vi "aft_LMS_Set_Memory.vi"(8 "error in":errorcluster, 10 "fixed-point LMS settings":T1, 11 "diagram":refnum<vi>) -> (0 "error out":errorcluster, 3 "diagram out":refnum<vi>)   [LabVIEW 2017, in "NI_AdaptiveFilter.lvlib"]
uses:
  <vilib>/addons/Adaptive Filters/NI_AdaptiveFilter.lvlib
  <vilib>/fxp/LVFixedPointRepBitsTypeDef.ctl
  <vilib>/rvi/ClientSDK/Core/Script/Memory/ProjectItem/Public/nirviPiMemoryType_ArbitrationOption.ctl
  <vilib>/rvi/DataTransferAndStorage/Container/Common/niFpgaContainerMemoryLatencyControl.ctl
  <vilib>/rvi/ClientSDK/Core/Script/Memory/ProjectItem/Private/nirviPiMemory_CommitLocal.vi
  <vilib>/rvi/ClientSDK/Core/Script/Memory/ProjectItem/Private/nirviPiMemory_SetArbitrationOptions.vi
  <vilib>/rvi/ClientSDK/Core/Script/Memory/ProjectItem/Private/nirviPiMemory_SetInitData2.vi
  <vilib>/rvi/ClientSDK/Core/Script/Memory/ProjectItem/Private/nirviPiMemory_SetSize.vi
  <vilib>/rvi/ClientSDK/Core/Script/Memory/ProjectItem/Private/nirviPiMemory_SetMemoryLatency.vi
  <vilib>/rvi/ClientSDK/Core/Script/Memory/ProjectItem/Private/nirviPiMemory_SetDataType2.vi
  <vilib>/rvi/ClientSDK/Core/Script/Memory/ProjectItem/Private/nirviPiMemory_OpenWithNodeRefnum.vi
  <vilib>/Utility/VariantDataType/VariantType.lvlib
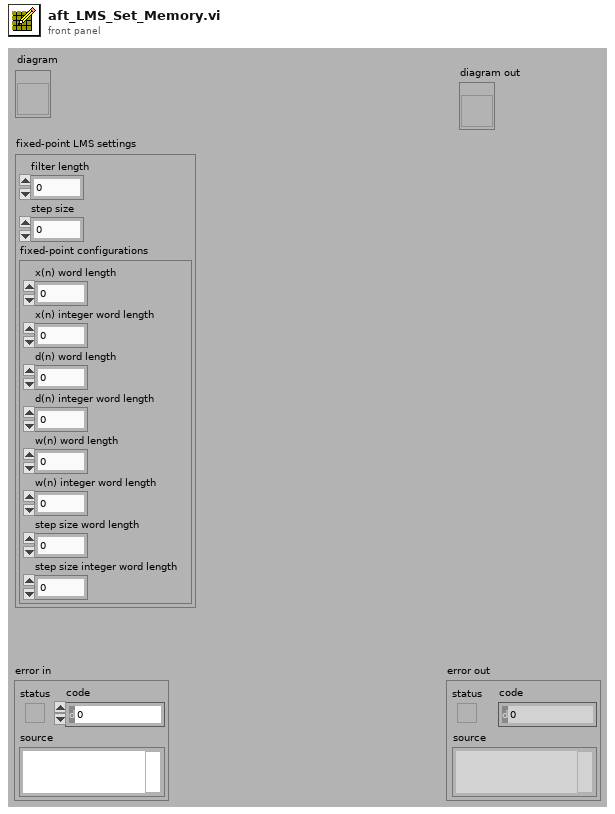
[diagram p1: front panel]
types:
  T1 = cluster{"filter length":i32, "step size":dbl, "fixed-point configurations":cluster{"x(n) word length":i32, "x(n) integer word length":i32, "d(n) word length":i32, "d(n) integer word length":i32, "w(n) word length":i32, "w(n) integer word length":i32, "step size word length":i32, "step size integer word length":i32}}
  T2 = typedef "LVFixedPointRepBitsTypeDef.ctl" = cluster{"Signed":bool, "Word Length":u32, "Integer Word Length":i32}
  T3 = typedef "nirviPiMemoryType_ArbitrationOption.ctl" = u16
  T4 = typedef "nirviPiMemory_State.ctl" = cluster{"Item":refnum<vi>, "Memory Block":T5, "Dirty":bool, "XNode":refnum<vi>, "Init Data String":string}
  T5 = typedef "niFpgaContainerState.ctl" = cluster{"displayName":string, "hardwareName":string, "dataType":T6, "elementTypeDescriptor":variant, "terminalTypeDescriptor":variant, "requestedNumberOfElements":u32, "memoryType":T7, "arbitrationForInterfaceA":T8, "numberOfElementsPerRead":u32, "arbitrationForInterfaceB":T8, "numberOfElementsPerWrite":u32, "VI_Defined":bool, "type":T9, "initializationParameters":T10, "disableOnOverflow/Underflow":bool, "interfaceConfiguration":T11, "controlLogic":T12, "actualNumberOfElements":u32, "dramSelection":string, "dramMaxOustandingRequests":i32, "dramIncludeByteEnables":bool, "dramGrantTime":u32, "fullEmulation":bool, "memoryInMultipleClockDomains":bool, "memoryLatency":T13}
  T6 = typedef "niFpgaDataTypeControl.ctl" = enum32{"Boolean", "I8", "I16", "I32", "I64", "U8", "U16", "U32", "U64", "FXP", "CustomControl", "SGL"}
  T7 = typedef "niFpgaContainerImplementationControl.ctl" = enum16{"Flip-Flops", "Look-Up Table", "Block Memory", "DRAM"}
  T8 = typedef "niFpgaContainerArbitrationOptionsControl.ctl" = enum16{"Always Arbitrate", "Arbitrate if Multiple Requestors Only", "Never Arbitrate"}
  T9 = typedef "niFpgaTransferTypeControl.ctl" = enum16{"Target-Scoped", "Host to Target - DMA", "Target to Host - DMA", "Peer to Peer Reader", "Peer to Peer Writer", "Bidirectional"}
  T10 = typedef "niFpgaContainerInitializationParameters.ctl" = cluster{"initialized":bool, "VI_Path":path, "initialData":variant}
  T11 = typedef "niFpgaMemoryInterfaceConfiguration.ctl" = enum16{"Read A-Write B", "Read A-Read B"}
  T12 = typedef "niFpgaFifoControlLogicControl.ctl" = enum16{"Slice Fabric", "Target Optimal", "Built-in"}
  T13 = typedef "niFpgaContainerMemoryLatencyControl.ctl" = u16
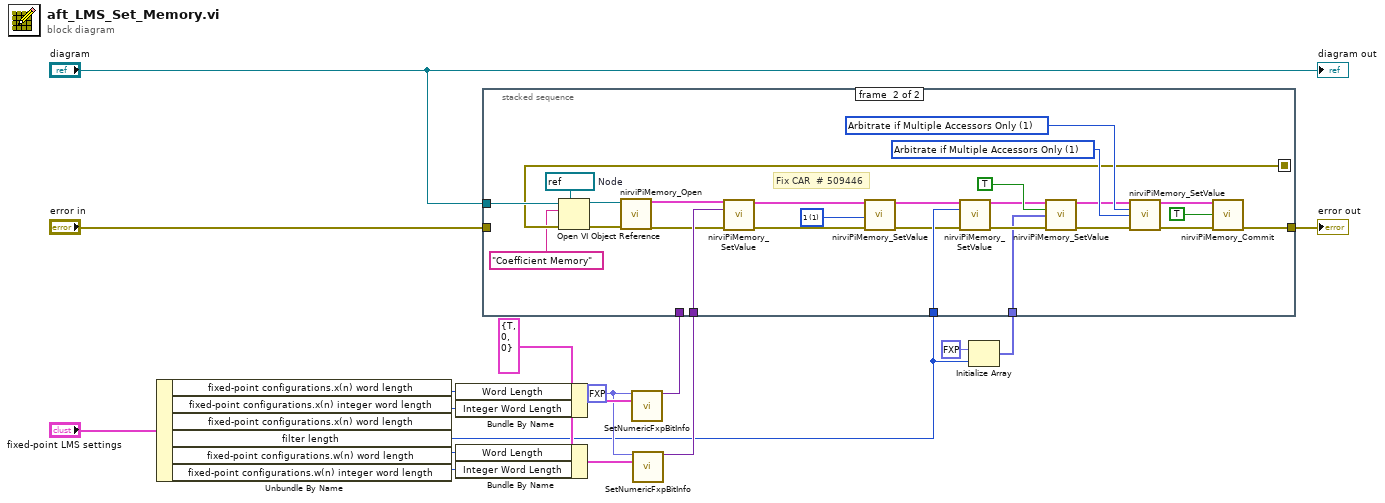
[diagram p0: block diagram]
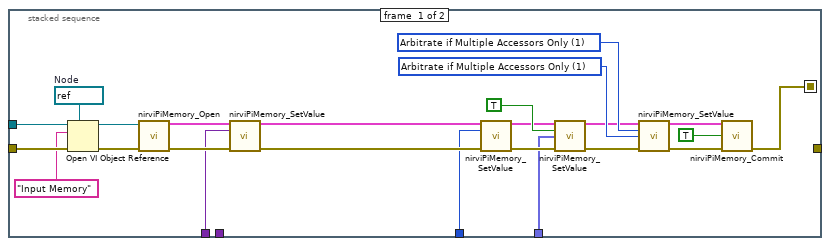
[diagram p2: hidden frame]
diagram:
  w4 = fxp<+,1,1> 0.0
  w9 = T2 {"Signed"=TRUE, "Word Length"=0, "Integer Word Length"=0} ("FxpRepresentation")
  n1 = Unbundle By Name("fixed-point LMS settings") -> ("fixed-point configurations.x(n) word length"=w13:i32, "fixed-point configurations.x(n) integer word length"=w12:i32, "filter length"=w1:i32, "fixed-point configurations.w(n) word length"=w8:i32, "fixed-point configurations.w(n) integer word length"=w7:i32)  [unwired: 1 out]
  n2 = Bundle By Name(cluster=w9, "Word Length"=w13, "Integer Word Length"=w12) -> (w11:T2)
  n3 = Bundle By Name(cluster=w9, "Word Length"=w8, "Integer Word Length"=w7) -> (w6:T2)
  n4 = call <vilib>:"SetNumericFxpBitInfo.vi"("Variant"=w4, "FxpRepresentation"=w11) -> ("Modified Variant"=w10:variant)  [unwired: 1 in, 12 out]
  n5 = call <vilib>:"SetNumericFxpBitInfo.vi"("Variant"=w4, "FxpRepresentation"=w6) -> ("Modified Variant"=w5:variant)  [unwired: 1 in, 12 out]
  n6 = Initialize Array(fxp<+,1,1> 0.0 ("y"), w1) -> (w2:fxp<+,1,1>[])
  n7 = stacked-sequence {
    seq-local: [w27 _] -> [_ w49]
    tunnel: w1 -> [w19 w57]
    tunnel: w5 -> [_ w58]
    tunnel: [_ w56] -> w17
    tunnel: "error in" -> [w22 _]
    tunnel: "diagram" -> [w23 w50]
    tunnel: w10 -> [w20 _]
    tunnel: w2 -> [w18 w47]
    frame #0 {
      w26 = refnum<vi> refnum  # Node
      w38 = T3 1 items=["Always Arbitrate", "Arbitrate if Multiple Accessors Only", "Never Arbitrate"] ("Read Arbitration")
      w37 = T3 1 items=["Always Arbitrate", "Arbitrate if Multiple Accessors Only", "Never Arbitrate"] ("Read Arbitration")
      n8 = Open VI Object Reference(7:w26, 8:w22, 10:"Input Memory" ("name/order"), 11:w23) -> (0:w25:errorcluster, 3:w24:refnum<vi>)
      n9 = call-poly <vilib>:"nirviPiMemory_Open.vi"("Local Fifo Node"=w24, "error in (no error)"=w25) -> ("Reference"=w28:T4, "error out"=w29:errorcluster)  [unwired: 12 out]
      n10 = call-poly <vilib>:"nirviPiMemory_SetValue.vi"("Reference"=w28, "Data Type"=w20, "error in (no error)"=w29) -> ("Reference"=w30:T4, "error out"=w31:errorcluster)  [unwired: 11 out]
      n11 = call-poly <vilib>:"nirviPiMemory_SetValue.vi"("Memory Reference"=w30, "Size"=w19, "error in (no error)"=w31) -> ("Memory Reference"=w33:T4, "error out"=w32:errorcluster)  [unwired: 11 out]
      n12 = call-poly <vilib>:"nirviPiMemory_SetValue.vi"("Memory Reference"=w33, "Init Block"=TRUE, "Init Data"=w18, "error in (no error)"=w32) -> ("Memory Reference"=w35:T4, "error out"=w36:errorcluster)  [unwired: 10 out]
      n13 = call-poly <vilib>:"nirviPiMemory_SetValue.vi"("Memory Reference"=w35, "Read Arbitration"=w37, "Write Arbitration"=w38, "error in (no error)"=w36) -> ("Memory Reference"=w39:T4, "error out"=w40:errorcluster)  [unwired: 10 out]
      n14 = call-poly <vilib>:"nirviPiMemory_Commit.vi"("Reference"=w39, "Close Reference?"=TRUE, "error in (no error)"=w40) -> ("error out"=w27:errorcluster)  [unwired: 12 out]
    }
    frame #1 {
      w46 = T13 1 items=["0", "1", "2", "3"] ("Memory Latency")
      w52 = refnum<vi> refnum  # Node
      w65 = T3 1 items=["Always Arbitrate", "Arbitrate if Multiple Accessors Only", "Never Arbitrate"] ("Read Arbitration")
      w64 = T3 1 items=["Always Arbitrate", "Arbitrate if Multiple Accessors Only", "Never Arbitrate"] ("Read Arbitration")
      # "Fix CAR  # 509446"
      n15 = Open VI Object Reference(7:w52, 8:w49, 10:"Coefficient Memory" ("name/order"), 11:w50) -> (0:w53:errorcluster, 3:w51:refnum<vi>)
      n16 = call-poly <vilib>:"nirviPiMemory_Open.vi"("Local Fifo Node"=w51, "error in (no error)"=w53) -> ("Reference"=w55:T4, "error out"=w54:errorcluster)  [unwired: 1 in, 11 out]
      n17 = call-poly <vilib>:"nirviPiMemory_SetValue.vi"("Reference"=w55, "Data Type"=w58, "error in (no error)"=w54) -> ("Reference"=w44:T4, "error out"=w45:errorcluster)  [unwired: 11 out]
      n18 = call-poly <vilib>:"nirviPiMemory_SetValue.vi"("Memory Reference in"=w44, "Memory Latency"=w46, "error in (no error)"=w45) -> ("Memory Reference out"=w43:T4, "error out"=w42:errorcluster)  [unwired: 11 out]
      n19 = call-poly <vilib>:"nirviPiMemory_SetValue.vi"("Memory Reference"=w43, "Size"=w57, "error in (no error)"=w42) -> ("Memory Reference"=w60:T4, "error out"=w59:errorcluster)  [unwired: 11 out]
      n20 = call-poly <vilib>:"nirviPiMemory_SetValue.vi"("Memory Reference"=w60, "Init Block"=TRUE, "Init Data"=w47, "error in (no error)"=w59) -> ("Memory Reference"=w62:T4, "error out"=w63:errorcluster)  [unwired: 10 out]
      n21 = call-poly <vilib>:"nirviPiMemory_SetValue.vi"("Memory Reference"=w62, "Read Arbitration"=w64, "Write Arbitration"=w65, "error in (no error)"=w63) -> ("Memory Reference"=w66:T4, "error out"=w67:errorcluster)  [unwired: 10 out]
      n22 = call-poly <vilib>:"nirviPiMemory_Commit.vi"("Reference"=w66, "Close Reference?"=TRUE, "error in (no error)"=w67) -> ("error out"=w56:errorcluster)  [unwired: 12 out]
    }
  }
  "error out" <- w17
  "diagram out" <- "diagram"
